vi "Tree_Sync_Open Items.vi"(8 "error in (no error)":errorcluster, 10 "All Tree Control Refs":refnum<vi>[](array[refnum]), 11 "Main Tree Control Ref":refnum<vi>) -> (0 "error out":errorcluster)   [LabVIEW 2023]
doc: "Synchronize open/closed tree items between main tree (master) and other tree refs in array."
panel:
  out "Open":bool[](array[boolean])
  out "Open Item Tags":string[](array[string])
  in  "Debug Tree":string[](tree)
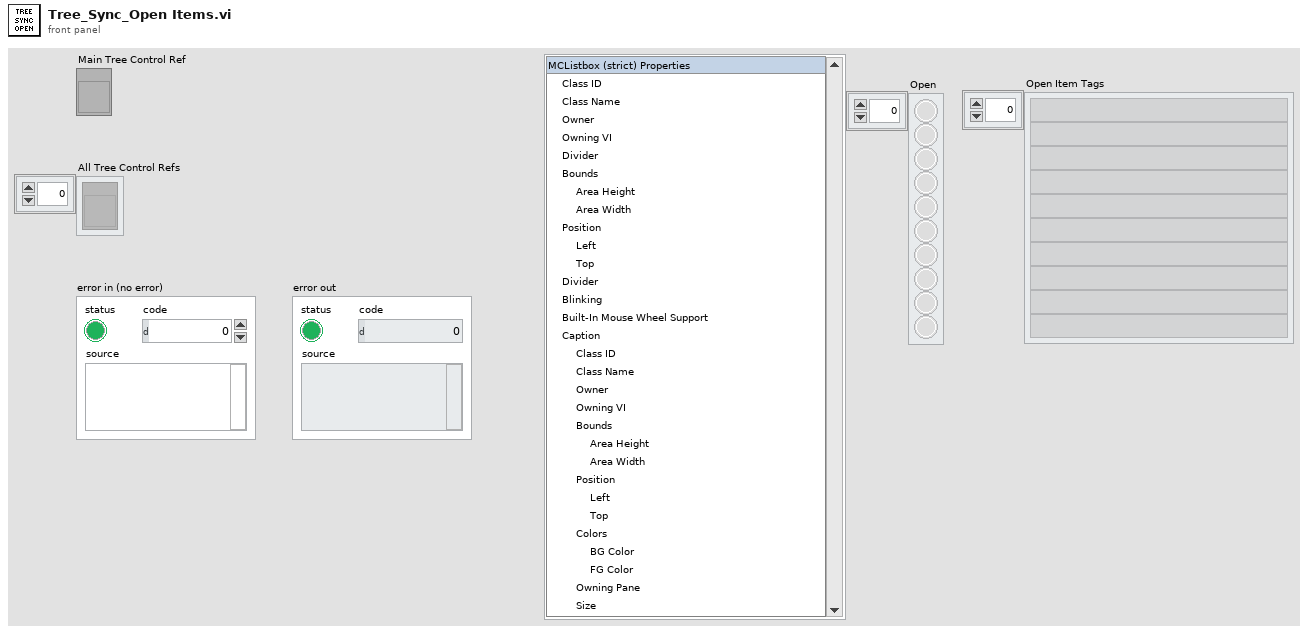
[diagram p1: front panel]
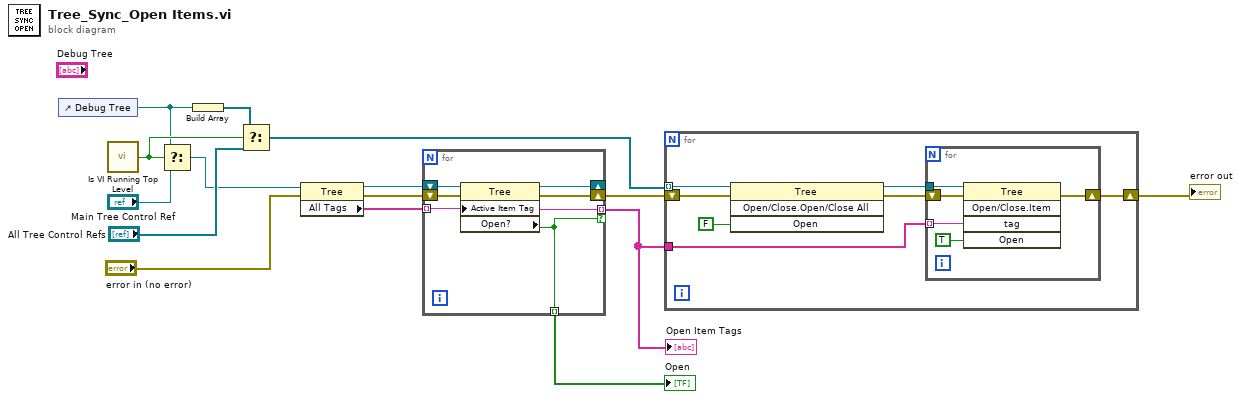
[diagram p0: block diagram]
diagram:
  n1 = control-ref of="Debug Tree"() -> (w9:refnum<vi>)
  n2 = call "Is VI Running Top Level.vi"() -> ("Top Level?"=w10:bool)  [unwired: 5 in]
  n3 = Select(t=w9, s=w10, f="Main Tree Control Ref") -> (s? t:f=w3:refnum<vi>)
  n4 = Build Array(w9) -> (w8:refnum<vi>[])
  n5 = Select(t=w8, s=w10, f="All Tree Control Refs") -> (s? t:f=w6:refnum<vi>[])
  n6 = property class="Tree"(reference=w3, error in="error in (no error)") -> (reference out=w15:refnum<vi>, error out=w13:errorcluster, "All Tags"=w5:string[])
  n7 = for {
    shift-right: [w17] -> _
    shift-left: w15 -> [w21]
    tunnel: w5 -> [w18] mode=indexing
    shift-right: [w19] -> w12
    shift-left: w13 -> [w20]
    tunnel: [w18] -> w2 mode=indexing if=w16
    tunnel: [w16] -> w1 mode=indexing
    n8 = property class="Tree"(reference=w21, error in=w20, "Active Item Tag"=w18) -> (reference out=w17:refnum<vi>, error out=w19:errorcluster, "Open?"=w16:bool)
  }
  "Open Item Tags" <- w2
  "Open" <- w1
  n9 = for {
    tunnel: w6 -> [w28] mode=indexing
    tunnel: w2 -> [w25]
    shift-right: [w23] -> w11
    shift-left: w12 -> [w24]
    n10 = invoke class="Tree" method="Open/Close.Open/Close All"(reference=w28, error in=w24, "Open"=FALSE ("Open?")) -> (reference out=w27:refnum<vi>, error out=w22:errorcluster)  [unwired: 1 in, 2 out]
    n11 = for {
      tunnel: w27 -> [w33]
      tunnel: w25 -> [w32] mode=indexing
      shift-right: [w31] -> w23
      shift-left: w22 -> [w30]
      n12 = invoke class="Tree" method="Open/Close.Item"(reference=w33, error in=w30, "tag"=w32, "Open"=TRUE ("Open?")) -> (error out=w31:errorcluster)  [unwired: 1 in, 4 out]
    }
  }
  "error out" <- w11
